vi "monitoreo.vi"() -> ()   [LabVIEW 2020]
uses:
  <vilib>/Instr/_visa.llb/VISA Configure Serial Port (Instr).vi
panel:
  in  "Boolean 3":bool
  out "error out":errorcluster
  in  "String 3":string
  out "String 2":string
  in  "Boolean 2":bool
  out "String":string
  in  "Boolean":bool
  in  "VISA resource name":refnum<visa-resource-name>
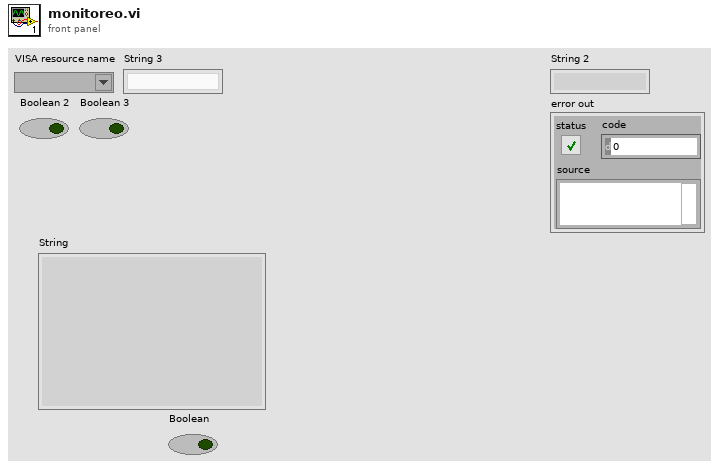
[diagram p1: front panel]
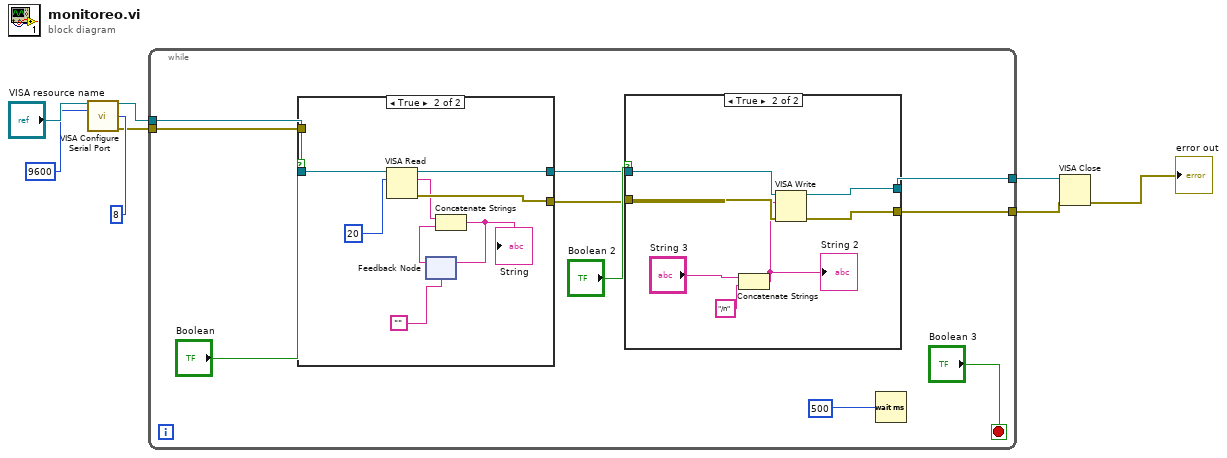
[diagram p0: block diagram]
diagram:
  n1 = call-poly "VISA Configure Serial Port"("VISA resource name"="VISA resource name", "baud rate (9600)"=9600, "data bits (8)"=8) -> ("VISA resource name out"=w5:refnum<visa-resource-name>, "error out"=w4:errorcluster)  [unwired: 11 in]
  n2 = while {
    tunnel: w5 -> [w16]
    tunnel: w4 -> [w12]
    tunnel: [w11] -> w3
    tunnel: [w10] -> w2
    stop <- "Boolean 3" stop-if-true
    n3 = case shown="True" "Boolean" {
      tunnel: w16 -> [w29 w36]
      tunnel: [w29 w35] -> w14
      tunnel: [w28 w34] -> w13
      tunnel: w12 -> [w28 _]
      frame False {
      }
      frame True {
        n4 = VISA Read(VISA resource name=w36, byte count=20) -> (VISA resource name out=w35:refnum<visa-resource-name>, read buffer=w33:string, error out=w34:errorcluster)  [unwired: 1 in, 1 out]
        n5 = feedback #1("") -> (w32:string)
        n6 = Concatenate Strings(w33, w32) -> (w31:string)
        "String" <- w31
        n7 = feedback-in #1(w31) -> ()
      }
    }
    n8 = case shown="True" "Boolean 2" {
      tunnel: w14 -> [w20 w27]
      tunnel: w13 -> [w19 w26]
      tunnel: [w19 w25] -> w10
      tunnel: [w20 w24] -> w11
      frame False {
      }
      frame True {
        n9 = Concatenate Strings("String 3", "/n") -> (w23:string)
        "String 2" <- w23
        n10 = VISA Write(VISA resource name=w27, write buffer=w23, error in (no error)=w26) -> (VISA resource name out=w24:refnum<visa-resource-name>, error out=w25:errorcluster)  [unwired: 1 out]
      }
    }
    n11 = Wait (ms)(milliseconds to wait=500) -> ()  [unwired: 1 out]
  }
  n12 = VISA Close(VISA resource name=w3, error in (no error)=w2) -> (error out=→"error out":errorcluster)
